vi "Switch Retrieve Key Array for Config.vi"(8 "error in (no error)":errorcluster, 10 "Key Array In":T6, 11 "Connection Refnum":T1) -> (0 "error out":errorcluster, 2 "Switch Test Parameters":T2, 3 "Connection Refnum":T1)   [LabVIEW 2011]
uses:
  ITK EXT/utils/keyedarr.llb/Keyed Array.ctl
  TypeDefs/Switch Test Parameters.ctl
  TypeDefs/Switch Stimulus Parameters.ctl
  TypeDefs/Switch Type.ctl
  TypeDefs/Switch Instrument Info.ctl
  Summitek EXT/ODBC/SQL Controls/Connection Refnum.ctl
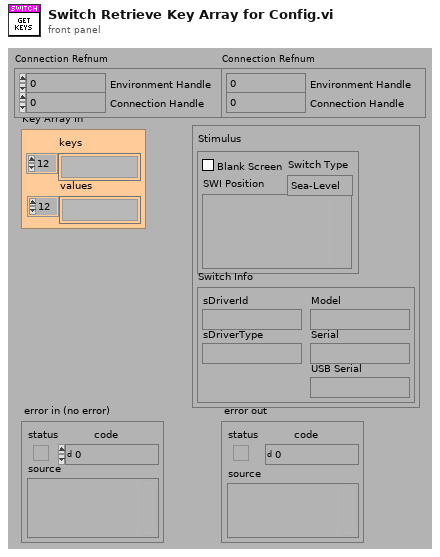
[diagram p1: front panel]
types:
  T1 = typedef "Connection Refnum.ctl" = cluster{"Environment Handle":i32, "Connection Handle":i32}
  T2 = typedef "Switch Test Parameters.ctl" = cluster{"Stimulus":T3, "Switch Info":T5}
  T3 = typedef "Switch Stimulus Parameters.ctl" = cluster{"Blank Screen":bool, "SWI Position":variant, "Switch Type":T4}
  T4 = typedef "Switch Type.ctl" = enum16{"Sea-Level", "Simulator", "SI-0206-SW", "SI-0309-SW", "SI-0310-SW", "Front End"}
  T5 = typedef "Switch Instrument Info.ctl" = cluster{"sDriverId":string, "sDriverType":string, "Model":string, "Serial":string, "USB Serial":string}
  T6 = typedef "Keyed Array.ctl" = cluster{"keys":string[], "values":string[]}
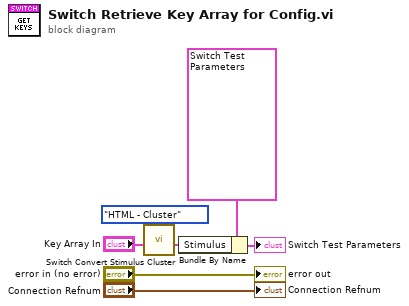
[diagram p0: block diagram]
diagram:
  n1 = call "Switch Convert Stimulus Cluster.vi"("Conversion"=enum16{"Cluster - HTML", "HTML - Cluster"}."HTML - Cluster", "Stimulus Key Array In"="Key Array In") -> ("Stimulus Cluster Out"=w3:T3)  [unwired: 5 in, 1 out]
  n2 = Bundle By Name(cluster=T2 {"Stimulus"={"Blank Screen"=FALSE, "SWI Position"=variant, "Switch Type"=enum."Simulator"}, "Switch Info"={"sDriverId"="", "sDriverType"="", "Model"="", "Serial"="", "USB Serial"=""}} ("DCA Test Parameters"), "Stimulus"=w3) -> (→"Switch Test Parameters":T2)
  "error out" <- "error in (no error)"
  "Connection Refnum" <- "Connection Refnum"
